vi "Output.vi"(8 "error in (no error)":errorcluster, 11 "Pump Calibration Config in":T1={"Settings"={"Cycle Period"=500.0, "Ismatech"={"VISA resource name"="", "Simulated?"=TRUE, "Pump Number"=1.0, "Reverse?"=FALSE}, "Masterflex"={"VISA resource name"="", "Simulated?"=TRUE, "Pump Number"=1.0, "Reverse?"=FALSE}, "Bronkhorst M13 Flow Meter"={"VISA resource name"="", "Simulated?"=TRUE}, "PID 2 Parameters"={"Input Device"=enum."Default", "Output Device"=enum."Default"}, "Bronkhorst M14"={"VISA resource name"="", "Simulated?"=FALSE}, "Tacmina Settings"={"Analog DAQ Task"="", "Digital DAQ Task"=""}, "KNF SIMDOS Settings"={"VISA resource name"="", "Simulated?"=TRUE}, "VICI M50 Settings"={"VISA resource name"="", "Simulated?"=TRUE, "Pump Letter"="", "Reverse?"=FALSE}, "FLOM Settings"={"VISA resource name"="", "Simulated?"=TRUE, "Pump Number"=0.0}, "Calibration Limits"={"Minimum (ml/min)"=0.0, "Maximum (ml/min)"=0.0, "Steps"=0.0}, "SSI PR Settings"={"VISA resource name"="", "Simulated?"=FALSE}}, "Flowmeter Output"=0.0, "Density"=0.0, "FL Temp"=0.0, "Speed %"=0.0, "File Refnum"=refnum, "Pump On?"=enum."Not Initialized"} {"Settings"."Masterflex"."Pump Number" min=1.0 max=20.0 step=1.0; "Settings"."Ismatech"."Pump Number" min=1.0 max=20.0 step=1.0}) -> (0 "error out":errorcluster, 3 "Pump Calibration Config Out":T1={"Settings"={"Cycle Period"=500.0, "Ismatech"={"VISA resource name"="", "Simulated?"=TRUE, "Pump Number"=1.0, "Reverse?"=FALSE}, "Masterflex"={"VISA resource name"="", "Simulated?"=TRUE, "Pump Number"=1.0, "Reverse?"=FALSE}, "Bronkhorst M13 Flow Meter"={"VISA resource name"="", "Simulated?"=TRUE}, "PID 2 Parameters"={"Input Device"=enum."Default", "Output Device"=enum."Default"}, "Bronkhorst M14"={"VISA resource name"="", "Simulated?"=FALSE}, "Tacmina Settings"={"Analog DAQ Task"="", "Digital DAQ Task"=""}, "KNF SIMDOS Settings"={"VISA resource name"="", "Simulated?"=TRUE}, "VICI M50 Settings"={"VISA resource name"="", "Simulated?"=TRUE, "Pump Letter"="", "Reverse?"=FALSE}, "FLOM Settings"={"VISA resource name"="", "Simulated?"=TRUE, "Pump Number"=0.0}, "Calibration Limits"={"Minimum (ml/min)"=0.0, "Maximum (ml/min)"=0.0, "Steps"=0.0}, "SSI PR Settings"={"VISA resource name"="", "Simulated?"=FALSE}}, "Flowmeter Output"=0.0, "Density"=0.0, "FL Temp"=0.0, "Speed %"=0.0, "File Refnum"=refnum, "Pump On?"=enum."Not Initialized"} {"Settings"."Masterflex"."Pump Number" min=1.0 max=20.0 step=1.0; "Settings"."Ismatech"."Pump Number" min=1.0 max=20.0 step=1.0})   [LabVIEW 2018, in "Calibration.lvlib" / "Engine.lvlib"]
uses:
  Engine.lvlib
  Pump Calibration Config.ctl
  Pfizer Timed Seq/Software/Ismatec ISM 831C/Controls/Ismatech Settings Cluster.ctl
  Pfizer Timed Seq/Software/Masterflex 7550-30/Controls/Settings Cluster.ctl
  Pfizer Timed Seq/Software/Bronkhorst M13 Flow Meter/Settings Cluster.ctl
  Pfizer Timed Seq/Software/Measure Instrument/PID Input Enum.ctl
  Pfizer Timed Seq/Software/Measure Instrument/PID 2 Output Enum.ctl
  Pfizer Timed Seq/Software/Mettler Toledo/Controls/Settings Cluster.ctl
  Pfizer Timed Seq/Software/Tacmina QI/Tacmina QI DAQ Setting.ctl
  Pfizer Timed Seq/Software/KNF Pump/Settings Cluster plus SIMDOS.ctl
  Pfizer Timed Seq/Software/VICI M50 Party Mode/Settings Cluster.ctl
  Pfizer Timed Seq/Software/FLOM Pump/Settings Cluster.ctl
  Pfizer Timed Seq/Software/SSI PR Class/SSI PR Settings Cluster.ctl
  Pfizer Timed Seq/Software/Ismatec ISM 831C/Ismatec ISM 831C.lvlib
  Pfizer Timed Seq/Software/Masterflex 7550-30/Masterflex 7550-30.lvlib
  Pfizer Timed Seq/Software/VICI M50 Party Mode/VICI M6 M50 Party Mode.lvlib
  Pfizer Timed Seq/Software/Tacmina QI/Tacmina QI.lvlib
  Pfizer Timed Seq/Software/KNF Pump/KNF SIMDOS.lvlib
  Pfizer Timed Seq/Software/FLOM Pump/FLOM Pump.lvlib
  Pfizer Timed Seq/Software/SSI PR Class/SSI PR Pump.lvlib
  Pfizer Timed Seq/Software/Mettler Toledo/Mettler Toledo.lvlib
  Pfizer Timed Seq/Software/Bronkhorst M13 Flow Meter/Bronkhorst M13 Flow Meter.lvlib
  Pfizer Timed Seq/Software/Calibration VIs/Calibration.lvlib
panel:
  # "Output Instruments"
  # "Input Instruments"
  # "Output Instruments"
  # "Input Instruments"
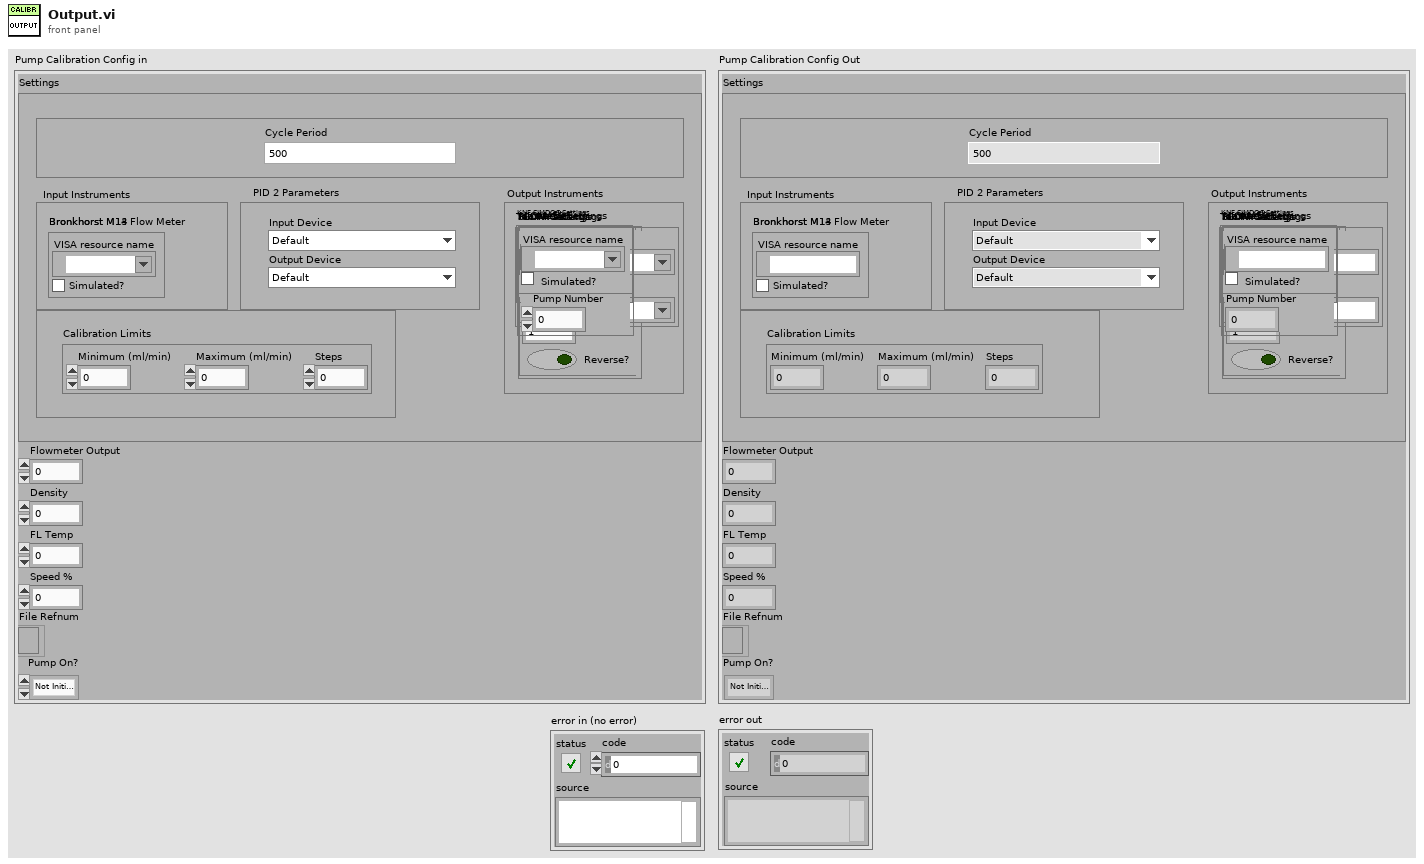
[diagram p1: front panel]
types:
  T1 = typedef "Calibration.lvlib/Pump Calibration Config.ctl" = cluster{"Settings":cluster{"Cycle Period":dbl, "Ismatech":T2, "Masterflex":T3, "Bronkhorst M13 Flow Meter":T4, "PID 2 Parameters":cluster{"Input Device":T5, "Output Device":T6}, "Bronkhorst M14":T7, "Tacmina Settings":T8, "KNF SIMDOS Settings":T9, "VICI M50 Settings":T10, "FLOM Settings":T11, "Calibration Limits":cluster{"Minimum (ml/min)":dbl, "Maximum (ml/min)":dbl, "Steps":dbl}, "SSI PR Settings":T12}, "Flowmeter Output":dbl, "Density":dbl, "FL Temp":dbl, "Speed %":dbl, "File Refnum":refnum<file>, "Pump On?":enum16{"Off", "On", "Not Initialized"}}
  T2 = typedef "Ismatec ISM 831C.lvlib/Ismatech Settings Cluster.ctl" = cluster{"VISA resource name":refnum<visa-resource-name>, "Simulated?":bool, "Pump Number":dbl, "Reverse?":bool}
  T3 = typedef "Masterflex 7550-30.lvlib/Settings Cluster.ctl" = cluster{"VISA resource name":refnum<visa-resource-name>, "Simulated?":bool, "Pump Number":dbl, "Reverse?":bool}
  T4 = typedef "Bronkhorst M13 Flow Meter.lvlib/Settings Cluster.ctl" = cluster{"VISA resource name":refnum<visa-resource-name>, "Simulated?":bool}
  T5 = typedef "PID Input Enum.ctl" = enum16{"Default", "Bronkhorst M13", "Bronkhorst M14", "Scale Rate of Change"}
  T6 = typedef "PID 2 Output Enum.ctl" = enum16{"Default", "Ismatec ISM 831C", "Masterflex 7550-30", "VICI", "Tacmina QI", "KNF SIMDOS", "ASIA Type C", "FLOM UI-22-11", "SSI PR"}
  T7 = typedef "Mettler Toledo.lvlib/Settings Cluster.ctl" = cluster{"VISA resource name":refnum<visa-resource-name>, "Simulated?":bool}
  T8 = typedef "Tacmina QI.lvlib/Tacmina QI DAQ Setting.ctl" = cluster{"Analog DAQ Task":refnum<k21>, "Digital DAQ Task":refnum<k21>}
  T9 = typedef "KNF SIMDOS.lvlib/Settings Cluster plus SIMDOS.ctl" = cluster{"VISA resource name":refnum<visa-resource-name>, "Simulated?":bool}
  T10 = typedef "VICI M6 M50 Party Mode.lvlib/Settings Cluster.ctl" = cluster{"VISA resource name":refnum<visa-resource-name>, "Simulated?":bool, "Pump Letter":string, "Reverse?":bool}
  T11 = typedef "FLOM Pump.lvlib/Settings Cluster.ctl" = cluster{"VISA resource name":refnum<visa-resource-name>, "Simulated?":bool, "Pump Number":dbl}
  T12 = typedef "SSI PR Pump.lvlib/SSI PR Settings Cluster.ctl" = cluster{"VISA resource name":refnum<visa-resource-name>, "Simulated?":bool}
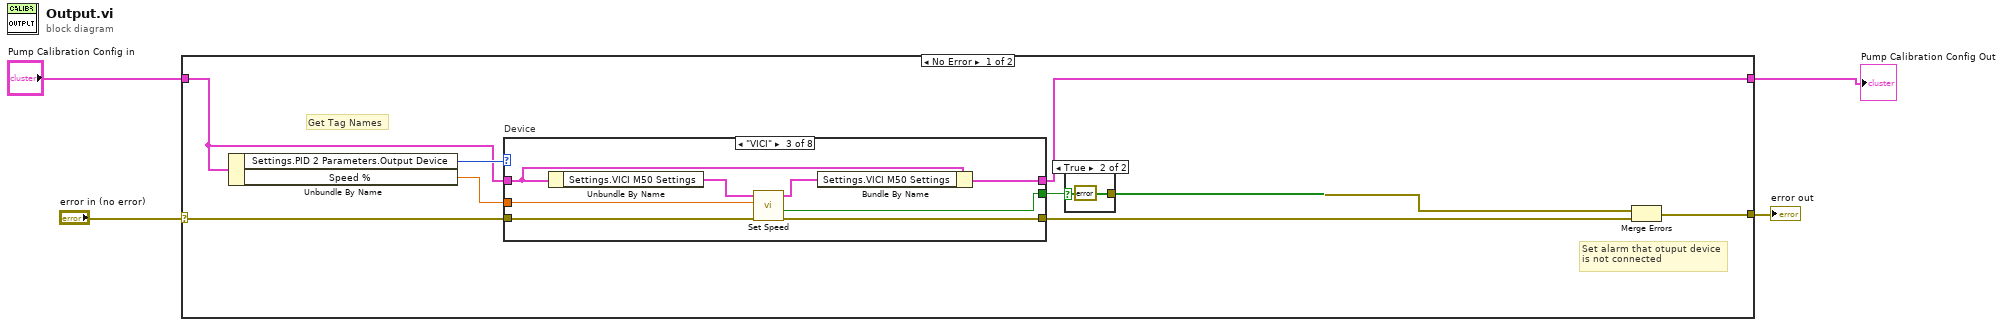
[diagram p0: block diagram]
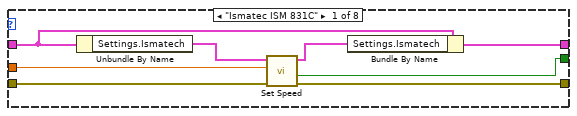
[diagram p2: hidden frame]
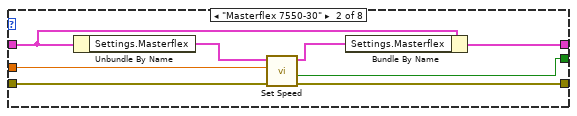
[diagram p3: hidden frame]
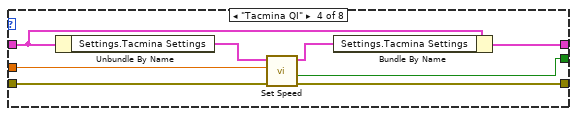
[diagram p4: hidden frame]
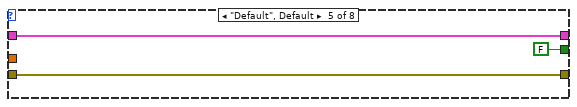
[diagram p5: hidden frame]
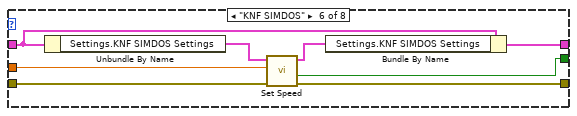
[diagram p6: hidden frame]
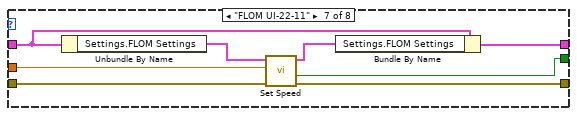
[diagram p7: hidden frame]
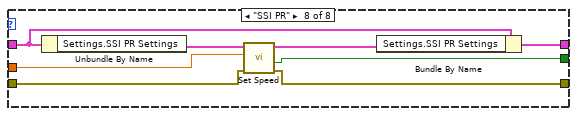
[diagram p8: hidden frame]
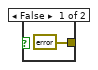
[diagram p9: hidden frame]
diagram:
  n1 = case shown="No Error" "error in (no error)" {
    selector: "error in (no error)" -> [w11 w76]
    tunnel: [w7 w76] -> w3
    tunnel: "Pump Calibration Config in" -> [w9 w75]
    tunnel: [w10 w75] -> w2
    frame No Error {
      # "Get Tag Names"
      # "Set alarm that otuput device\nis not connected"
      n2 = Unbundle By Name(w9) -> ("Settings.PID 2 Parameters.Output Device"=w13:T6, "Speed %"=w12:dbl)
      n3 = case "Device" shown="\"VICI\"" w13 {
        tunnel: w12 -> [w15 w23 w36 w44 _ w56 w60 w71]
        tunnel: w11 -> [w21 w25 w35 w43 w47 w54 w61 w70]
        tunnel: [w20 w24 w34 w42 w47 w51 w57 w69] -> w6
        tunnel: w9 -> [w19 w29 w31 w39 w48 w53 w62 w68]
        tunnel: [w16 w28 w33 w41 w48 w49 w59 w66] -> w10
        tunnel: [w14 w22 w30 w38 FALSE ("Connection Error") w50 w58 w65] -> w8
        frame "Ismatec ISM 831C" {
          n4 = Unbundle By Name(w19) -> ("Settings.Ismatech"=w18:T2)
          n5 = call "Set Speed.vi"("error in (no error)"=w21, "Speed (%)"=w15, "Ismatech Settings"=w18) -> ("error out"=w20:errorcluster, "Connection Error"=w14:bool, "Ismatech Settings"=w17:T2)  [unwired: 6 in]
          n6 = Bundle By Name(cluster=w19, "Settings.Ismatech"=w17) -> (w16:T1)
        }
        frame "Masterflex 7550-30" {
          n7 = Unbundle By Name(w29) -> ("Settings.Masterflex"=w27:T3)
          n8 = call "Set Speed.vi"("error in (no error)"=w25, "speed"=w23, "Masterflex Settings in"=w27) -> ("error out"=w24:errorcluster, "Connection Error"=w22:bool, "Masterflex Settings out"=w26:T3)  [unwired: 6 in]
          n9 = Bundle By Name(cluster=w29, "Settings.Masterflex"=w26) -> (w28:T1)
        }
        frame "VICI" {
          n10 = Unbundle By Name(w31) -> ("Settings.VICI M50 Settings"=w37:T10)
          n11 = call "Set Speed.vi"("error in (no error)"=w35, "speed"=w36, "VICI Settings"=w37) -> ("error out"=w34:errorcluster, "Connection Error"=w30:bool, "VICI Settings"=w32:T10)  [unwired: 6 in]
          n12 = Bundle By Name(cluster=w31, "Settings.VICI M50 Settings"=w32) -> (w33:T1)
        }
        frame "Tacmina QI" {
          n13 = Unbundle By Name(w39) -> ("Settings.Tacmina Settings"=w45:T8)
          n14 = call "Set Speed.vi"("error in"=w43, "Pump %"=w44, "Tacmina Settings in"=w45) -> ("error out"=w42:errorcluster, "Connection Error"=w38:bool, "Tacmina Settings out"=w40:T8)  [unwired: 6 in]
          n15 = Bundle By Name(cluster=w39, "Settings.Tacmina Settings"=w40) -> (w41:T1)
        }
        frame "Default", Default {
        }
        frame "KNF SIMDOS" {
          n16 = Unbundle By Name(w53) -> ("Settings.KNF SIMDOS Settings"=w55:T9)
          n17 = call "Set Speed.vi"("error in (no error)"=w54, "FlowRate"=w56, "KNF Settings"=w55) -> ("error out"=w51:errorcluster, "Connection Error"=w50:bool, "KNF Settings"=w52:T9)  [unwired: 6 in]
          n18 = Bundle By Name(cluster=w53, "Settings.KNF SIMDOS Settings"=w52) -> (w49:T1)
        }
        frame "FLOM UI-22-11" {
          n19 = Unbundle By Name(w62) -> ("Settings.FLOM Settings"=w64:T11)
          n20 = call "Set Speed.vi"("error in (no error)"=w61, "speed"=w60, "FLOM Settings in"=w64) -> ("error out"=w57:errorcluster, "Connection Error"=w58:bool, "FLOM Settings out"=w63:T11)  [unwired: 6 in]
          n21 = Bundle By Name(cluster=w62, "Settings.FLOM Settings"=w63) -> (w59:T1)
        }
        frame "SSI PR" {
          n22 = Unbundle By Name(w68) -> ("Settings.SSI PR Settings"=w72:T12)
          n23 = call "Set Speed.vi"("error in (no error)"=w70, "speed (ml/min)"=w71, "SSI PR Settings"=w72) -> ("error out"=w69:errorcluster, "Connection Error"=w65:bool, "SSI PR Settings"=w67:T12)  [unwired: 6 in]
          n24 = Bundle By Name(cluster=w68, "Settings.SSI PR Settings"=w67) -> (w66:T1)
        }
      }
      n25 = case shown="True" w8 {
        tunnel: [errorcluster {"status"=FALSE, "code"=0, "source"=""} ("error constant") errorcluster {"status"=TRUE, "code"=2, "source"="Output Error"} ("error constant")] -> w5
        frame False {
        }
        frame True {
        }
      }
      n26 = Merge Errors(w5, w6) -> (w7:errorcluster)
    }
    frame Error {
    }
  }
  "error out" <- w3
  "Pump Calibration Config Out" <- w2
